vi "unpack_pv.vi"(10 "payload_size":u32, 11 "payload":u64) -> (0 "height":u16, 1 "width":u16, 2 "metadata":T1, 3 "image":u32[][](array[numeric]), 4 "error":bool)   [LabVIEW 2023]
panel:
  in  "pv_metadata":T1
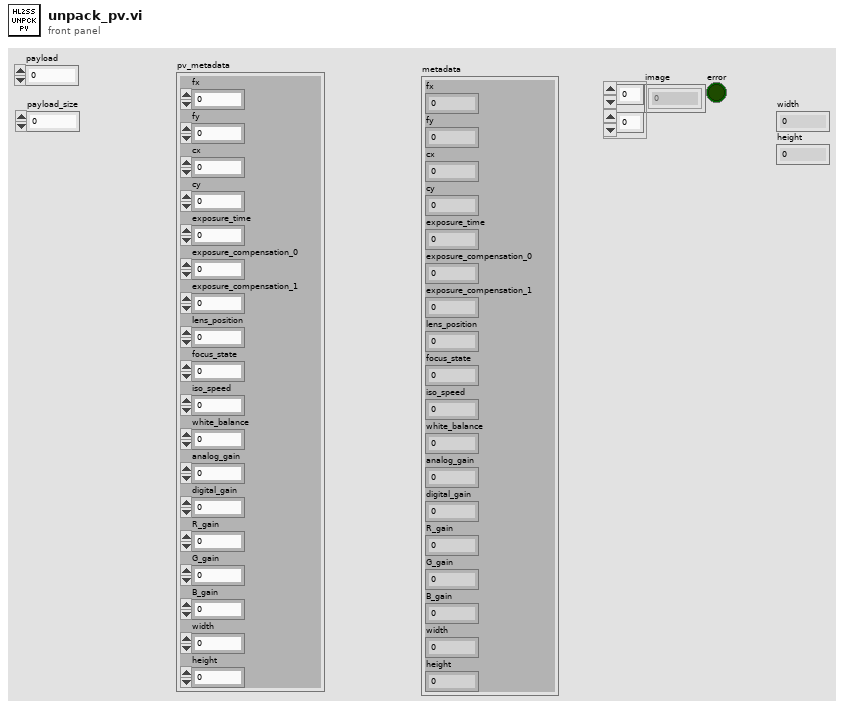
[diagram p1: front panel]
types:
  T1 = cluster{"fx":sgl, "fy":sgl, "cx":sgl, "cy":sgl, "exposure_time":u64, "exposure_compensation_0":u64, "exposure_compensation_1":u64, "lens_position":u32, "focus_state":u32, "iso_speed":u32, "white_balance":u32, "analog_gain":sgl, "digital_gain":sgl, "R_gain":sgl, "G_gain":sgl, "B_gain":sgl, "width":u16, "height":u16}
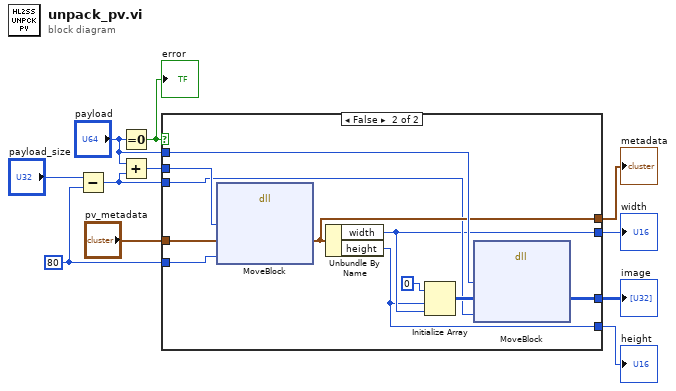
[diagram p0: block diagram]
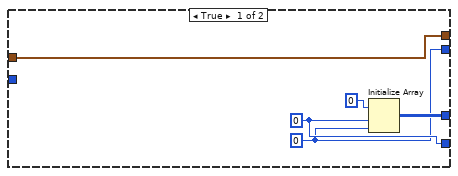
[diagram p2: hidden frame]
diagram:
  w5 = u64 80 ("size")
  n1 = Subtract(x="payload_size", y=w5) -> (x-y=w3:u64)
  n2 = Equal To 0?(x="payload") -> (x = 0?=w6:bool)
  "error" <- w6
  n3 = Add(x="payload", y=w3) -> (x+y=w11:u64)
  n4 = case shown="False" w6 {
    tunnel: "payload" -> [_ w27]
    tunnel: w11 -> [_ w26]
    tunnel: w5 -> [_ w25]
    tunnel: "pv_metadata" -> [w16 w24]
    tunnel: [w14 w23] -> w9
    tunnel: [w16 w20] -> w8
    tunnel: w3 -> [_ w19]
    tunnel: [w12 w18] -> w2
    tunnel: [w13 w17] -> w1
    frame True {
      w12 = 0 ("dimension size")
      w13 = 0 ("dimension size")
      n5 = Initialize Array(u32 0, w13, w12) -> (w14:u32[][])
    }
    frame False {
      n6 = dll-call lib="LabVIEW" fn="MoveBlock"("ps"=w26, "pd"=w24, "size"=w25) -> ("pd"=w20:T1)  [unwired: 6 in, 2 out]
      n7 = Unbundle By Name(w20) -> ("width"=w18:u16, "height"=w17:u16)
      n8 = Initialize Array(u32 0, w17, w18) -> (w21:u32[][])
      n9 = dll-call lib="LabVIEW" fn="MoveBlock"("ps"=w27, "pd"=w21, "size"=w19) -> ("pd"=w23:u32[][])  [unwired: 6 in, 2 out]
    }
  }
  "image" <- w9
  "metadata" <- w8
  "width" <- w2
  "height" <- w1
